vi "PositionSpeedTest_Create.vi"(0 "reference in":refnum<class "PositionSpeedTest.lvclass">, 2 "Engine":bool, 3 "Dyno":bool, 5 "error in (no error)":errorcluster) -> (14 "reference out":refnum<class "PositionSpeedTest.lvclass">, 19 "error out":errorcluster)   [LabVIEW 2024, in "PositionSpeedTest.lvclass"]
uses:
  PositionSpeedTest.lvclass
  C:/Users/burakkorkmaz/Desktop/Leveling/labview-desing-patterns/Template Method Pattern/Test_class/Test.lvclass
  PositionSpeedTest.lvclass/PositionSpeedTest.ctl
  Test_class/Test.lvclass
panel:
  # "Connector Pane"
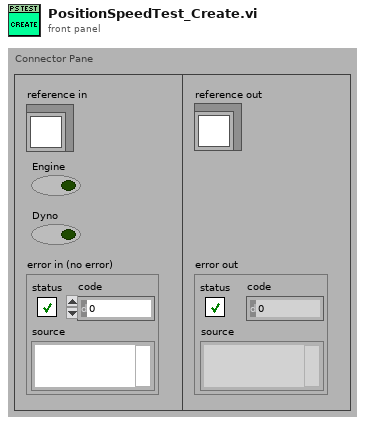
[diagram p1: front panel]
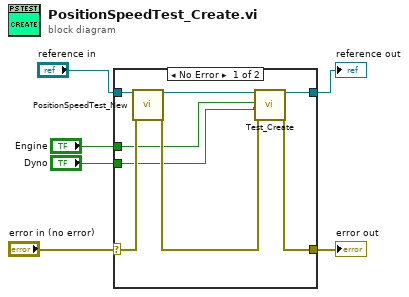
[diagram p0: block diagram]
diagram:
  n1 = case shown="No Error" "error in (no error)" {
    selector: "error in (no error)" -> [w13 w16]
    tunnel: [w9 w16] -> w5
    tunnel: "reference in" -> [w14 w15]
    tunnel: [w10 w15] -> w3
    tunnel: "Engine" -> [w8 _]
    tunnel: "Dyno" -> [w7 _]
    frame No Error {
      n2 = call "PositionSpeedTest_New.vi"("reference in"=w14, "error in (no error)"=w13) -> ("reference out"=w12:refnum<class "PositionSpeedTest.lvclass">, "error out"=w11:errorcluster)  [unwired: 14 in, 2 out]
      n3 = call "Test_Create.vi"("reference in"=w12, "Engine"=w8, "Dyno"=w7, "error in (no error)"=w11) -> ("reference out"=w10:refnum<class "PositionSpeedTest.lvclass">, "error out"=w9:errorcluster)  [unwired: 14 in]
    }
    frame Error {
    }
  }
  "error out" <- w5
  "reference out" <- w3
